vi "niDTS BT Tx Test UTIL Convert Framework Handle.vi"(9 "error in":errorcluster, 10 "InstDriver Handle":T2) -> (1 "error out":errorcluster, 2 "niRfsaBT":T1)   [LabVIEW 2015, in "niDTS BT.lvlib"]
uses:
  niDTS BT.lvlib
  RiviInstDriver/InstDriver/Includes/niInstDriver INC Handle.ctl
  RiviInstDriver/InstDriver/Objects/InstDriver.lvclass
  RiviInstDriver/niRfsaBT/Includes/niRfsaBt INC Handle.ctl
  RiviInstDriver/niRfsaBT/Objects/niRfsaBt.lvclass
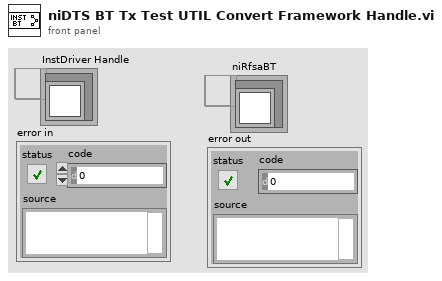
[diagram p1: front panel]
types:
  T1 = typedef "niRfsaBt.lvclass/niRfsaBT INC Handle.ctl" = refnum<data-value>
  T2 = typedef "InstDriver.lvclass/niInstDriver INC Handle.ctl" = refnum<data-value>
  T3 = typedef "niRfsaBT.lvclass/niRfsaBT INC Handle.ctl" = refnum<data-value>
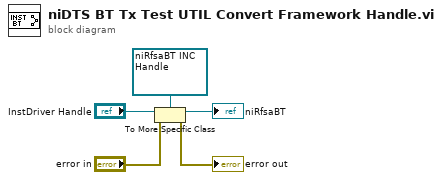
[diagram p0: block diagram]
diagram:
  n1 = To More Specific Class(target class=T3 refnum ("niRfsaBT"), reference="InstDriver Handle", error in="error in") -> (specific class reference=→"niRfsaBT":T3, error out=→"error out":errorcluster)
